vi "relative-file-path-finder.vi"() -> (0 "Config File":path)   [LabVIEW 2024]
panel:
  out "Project Folder":path
  out "current VI's path":path
  out "Current VI's folder":path
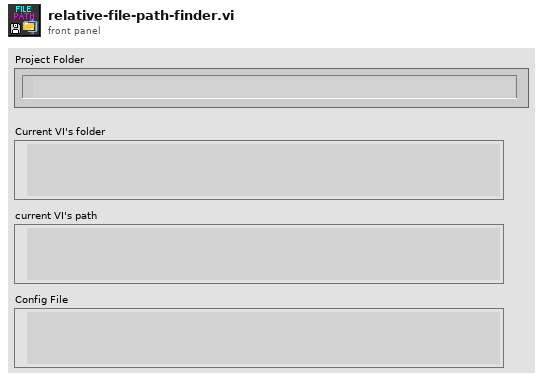
[diagram p1: front panel]
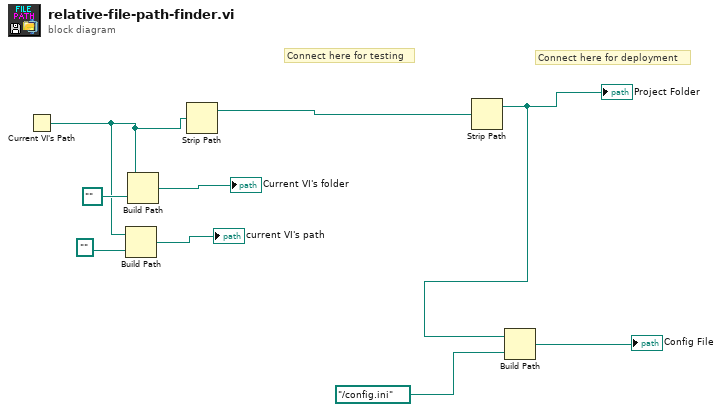
[diagram p0: block diagram]
diagram:
  # "Connect here for deployment"
  # "Connect here for testing"
  n1 = Current VI's Path() -> (path=w4:path)
  n2 = Build Path(base path=w4, name or relative path=path "") -> (appended path=→"current VI's path":path)
  n3 = Build Path(base path=w4, name or relative path=path "..") -> (appended path=→"Current VI's folder":path)
  n4 = Strip Path(path=w4) -> (stripped path=w3:path)  [unwired: 1 out]
  n5 = Strip Path(path=w3) -> (stripped path=w1:path)  [unwired: 1 out]
  "Project Folder" <- w1
  n6 = Build Path(base path=w1, name or relative path=path "../config.ini") -> (appended path=→"Config File":path)
